vi "SoundRead.vi"() -> ()   [LabVIEW 2015]
uses:
  <vilib>/sound2/lvsound2.llb/Sound Data Format.ctl
  <vilib>/sound2/lvsound2.llb/Sampling Mode.ctl
  <vilib>/sound2/lvsound2.llb/Sound Output Write (DBL).vi
  <vilib>/sound2/lvsound2.llb/Sound Input Read (DBL).vi
panel:
  out "Waveform Chart":waveform(dbl)[](graph)
  in  "stop":bool
  in  "data":waveform(dbl)[](array[waveform])
  in  "Output Device ID":u32
  in  "sound format":T1={"sample rate (S/s)"=22050.0, "number of channels"=2, "bits per sample"=16}
  in  "Input Device ID":u32
  in  "number of samples/ch":i32=100000
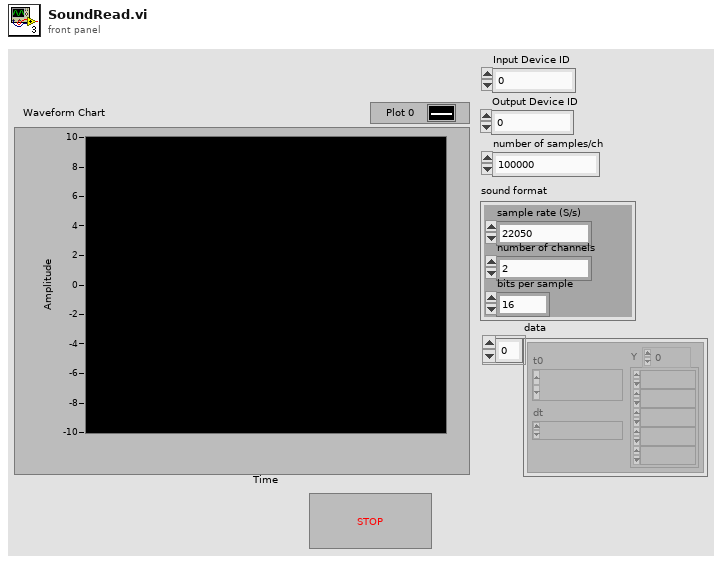
[diagram p1: front panel]
types:
  T1 = typedef "Sound Data Format.ctl" = cluster{"sample rate (S/s)":dbl, "number of channels":i32, "bits per sample":i32}
  T2 = typedef "Sampling Mode.ctl" = i32
  T3 = typedef "Sound Output Task ID.ctl" = u32
  T4 = typedef "Sound Input Task ID.ctl" = u32
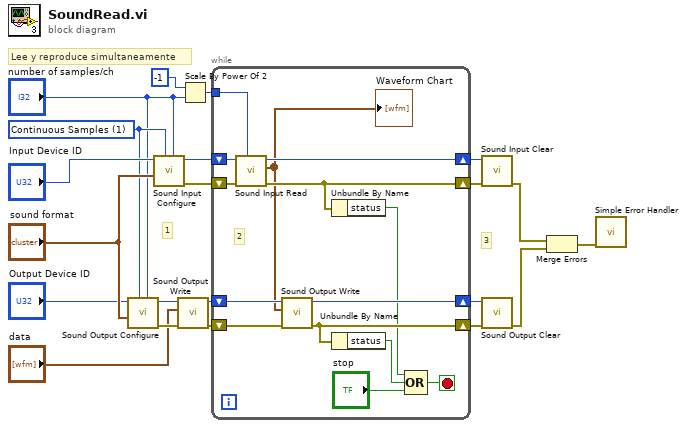
[diagram p0: block diagram]
diagram:
  w19 = T2 1 items=["Finite Samples", "Continuous Samples"] ("sample mode")
  # "3"
  # "Lee y reproduce simultaneamente"
  # "1"
  n1 = call <vilib>:"Sound Output Configure.vi"("number of samples/ch"="number of samples/ch", "sample mode"=w19, "sound format"="sound format", "device ID"="Output Device ID") -> ("error out"=w12:errorcluster, "task ID"=w11:T3)  [unwired: 6 in]
  n2 = call <vilib>:"Sound Input Configure.vi"("number of samples/ch"="number of samples/ch", "sample mode"=w19, "sound format"="sound format", "device ID"="Input Device ID") -> ("error out"=w13:errorcluster, "task ID"=w14:T4)  [unwired: 6 in]
  n3 = call-poly <vilib>:"Sound Output Write.vi"("error in (no error)"=w12, "data"="data", "task ID"=w11) -> ("error out"=w8:errorcluster, "task ID out"=w9:T3)  [unwired: 7 in]
  n4 = Scale By Power Of 2(n=i16 -1, x="number of samples/ch") -> (x*2^n=w15:i32)
  n5 = while {
    tunnel: w15 -> [w33]
    shift-right: [w30] -> w6
    shift-left: w14 -> [w34]
    shift-right: [w29] -> w7
    shift-left: w13 -> [w35]
    shift-right: [w28] -> w4
    shift-left: w9 -> [w31]
    shift-right: [w27] -> w5
    shift-left: w8 -> [w32]
    stop <- w24 stop-if-true
    # "2"
    n6 = call-poly <vilib>:"Sound Input Read.vi"("number of samples/ch"=w33, "error in (no error)"=w35, "task ID"=w34) -> ("error out"=w29:errorcluster, "data"=w23:waveform(dbl)[], "task ID out"=w30:T4)  [unwired: 6 in]
    "Waveform Chart" <- w23
    n7 = call-poly <vilib>:"Sound Output Write.vi"("error in (no error)"=w32, "data"=w23, "task ID"=w31) -> ("error out"=w27:errorcluster, "task ID out"=w28:T3)  [unwired: 7 in]
    n8 = Unbundle By Name(w29) -> ("status"=w22:bool)
    n9 = Unbundle By Name(w27) -> ("status"=w26:bool)
    n10 = Compound Arithmetic op=OR(w22, w26, "stop") -> (w24:bool)
  }
  n11 = call <vilib>:"Sound Input Clear.vi"("error in (no error)"=w7, "task ID"=w6) -> ("error out"=w2:errorcluster)  [unwired: 9 in]
  n12 = call <vilib>:"Sound Output Clear.vi"("error in (no error)"=w5, "task ID"=w4) -> ("error out"=w1:errorcluster)  [unwired: 9 in]
  n13 = Merge Errors(w2, w1) -> (w3:errorcluster)
  n14 = call <vilib>:"Simple Error Handler.vi"("error in (no error)"=w3) -> ()  [unwired: 4 in, 5 out]
